vi "start_multipart_post_request.vi"(7 "MultipartForm":refnum<class "MultipartForm.lvclass">, 8 "error in (no error)":errorcluster, 9 "Headers in":refnum<class "Headers.lvclass">, 10 "url":string, 11 "Client in":refnum<class "Client.lvclass">) -> (0 "error out":errorcluster, 2 "Request":refnum<class "Request.lvclass">, 3 "Client out":refnum<class "Client.lvclass">)   [LabVIEW 2020, in "reqwest.lvlib" / "Client.lvclass"]
uses:
  Client.lvclass
  Request/Request.lvclass
  MultipartForm/MultipartForm.lvclass
  Headers/Headers.lvclass
  Types/http_method_enum.ctl
  RequestBuilder/RequestBuilder.lvclass
  reqwest.lvlib
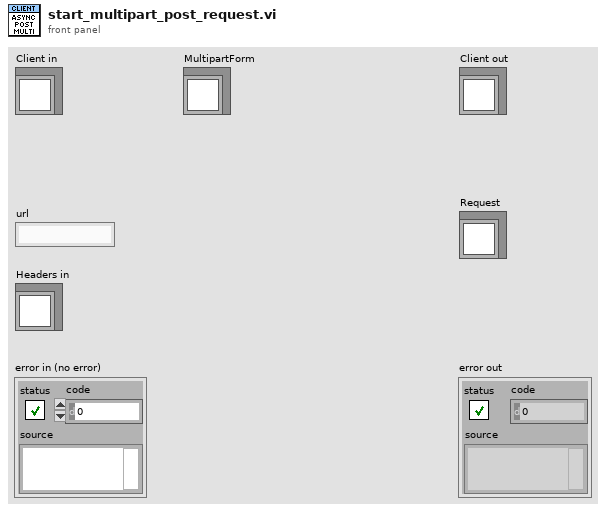
[diagram p1: front panel]
types:
  T1 = typedef "reqwest.lvlib/http_method_enum.ctl" = enum8{"<select>", "GET", "POST", "PUT", "DELETE", "HEAD", "OPTIONS", "CONNECT", "PATCH", "TRACE"}
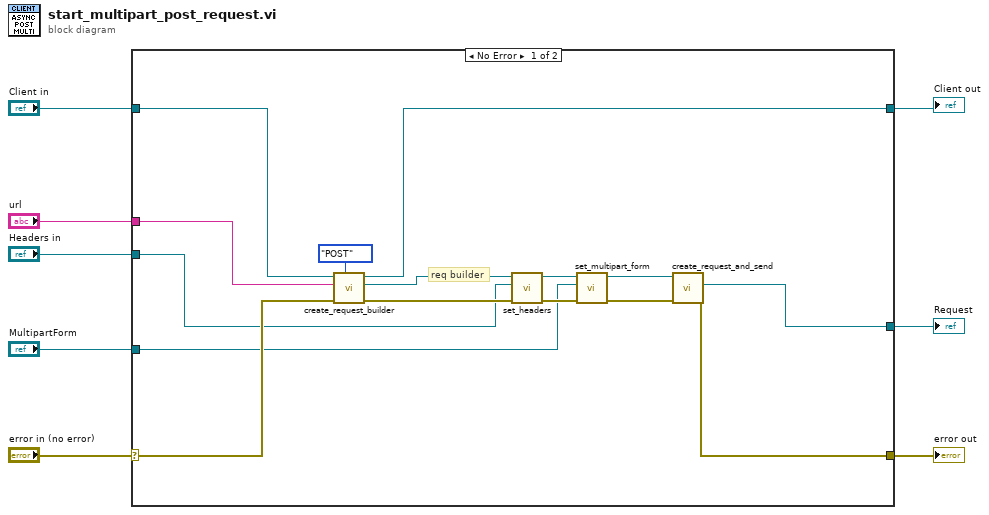
[diagram p0: block diagram]
diagram:
  n1 = case shown="No Error" "error in (no error)" {
    selector: "error in (no error)" -> [w19 w24]
    tunnel: "Client in" -> [w21 w25]
    tunnel: [w17 _] -> w6
    tunnel: [w18 w24] -> w4
    tunnel: [w22 w25] -> w5
    tunnel: "url" -> [w20 _]
    tunnel: "MultipartForm" -> [w9 _]
    tunnel: "Headers in" -> [w14 _]
    frame No Error {
      # "req builder"
      n2 = call "create_request_builder.vi"("HTTP Method"=http_method_enum."POST", "error in (no error)"=w19, "url"=w20, "Client in"=w21) -> ("error out"=w15:errorcluster, "RequestBuilder out"=w16:refnum<class "RequestBuilder.lvclass">, "Client out"=w22:refnum<class "Client.lvclass">)  [unwired: 5 in]
      n3 = call "set_headers.vi"("error in (no error)"=w15, "Headers"=w14, "obj in"=w16) -> ("error out"=w11:errorcluster, "obj out"=w13:refnum<class "RequestBuilder.lvclass">)  [unwired: 6 in, 1 out]
      n4 = call "set_multipart_form.vi"("error in (no error)"=w11, "MultipartForm"=w9, "RequestBuilder in"=w13) -> ("error out"=w10:errorcluster, "RequestBuilder out"=w12:refnum<class "RequestBuilder.lvclass">)  [unwired: 6 in, 1 out]
      n5 = call "create_request_and_send.vi"("error in"=w10, "obj in"=w12) -> ("error out"=w18:errorcluster, "request"=w17:refnum<class "Request.lvclass">)  [unwired: 7 in, 1 out]
    }
    frame Error {
    }
  }
  "error out" <- w4
  "Request" <- w6
  "Client out" <- w5
